vi "X-_Write.vi"(1 "Channel Name":string, 4 "Iteration No":i32, 6 "String to write":string, 7 "Port Name":string, 8 "Value":dbl format="%.2f", 9 "COMMAND":T1, 11 "Address":u8) -> (0 "Good Echo":bool)   [LabVIEW 2010]
uses:
  X-_commands.ctl
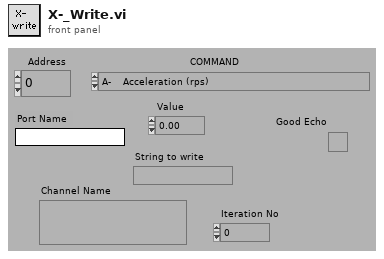
[diagram p1: front panel]
types:
  T1 = typedef "X-_commands.ctl" = enum16{"A-    Acceleration (rps)", "B-    Buffer Status", "C-    Continue", "CG-  Correction Gain", "CR-  Cariage Return", "D-    Distance (pulses)", "DB-  Dead Band (encoder steps)", "DW- Deadband Window (encoder steps)", "E-    Enable Communications", "ER-  Encoder Resolution (steps/rev)", "F-    Disable Communications", "FS-  Encoder Functions Report", "FSA- Incremental/Absolute (0/1)", "FSB- Motor/Encoder Step Mode (0/1)", "FSC- Enable/Disable Position Maint. (1/0)", "FSD- Stop/Continue on Stall (1/0)", "FSE- Activate o/p1 on Stall (1/0)", "FSF- Stop Motion on Trig3 (1/0)", "FSG- Activate o/p2 in Deadband (1/0)", "FSH- Enable Stall Detect (1/0)", "G- Go", "GH- Go Home and Zero (+/-V)", "^H- Delete ", "H- Direction Reverse/CCW/CW (0,1,2)", "IS- Input Status", "K- Kill", "L- Loop (n)", "LD- Limit DISABLE (0-none,1-CW,2-CCW,3-Both)", "LF- Line Feed", "MC- Mode Continuous", "MN- Mode Normal", "MPA- Motor Postion Absolute", "MPI- Motor Position Incremental", "MR- Motor Resolution (Drive Steps/rev)", "N- End of Loop", "O- Output (00,01,10,11)", "OS- Report Homing Setup", "OSA- NO/NC Limits (1/0)", "OSB- Back Up to Home/Edge? (0/1)", "OSC- NO/NC Home Switch (1/0)", "OSD- Enable Encoder Z for Home (0/1)", "OSH- Reference Edge for Home CW/CCW (0/1)", "PR- Report ABSOLUTE Position", "PS- Pause until Continue", "PX- Report Absolute ENCODER Position", "PZ- Zero Absolute Counter", "\"- Quote (17 ASCII +Space)", "Q- Enter/Exit Velocity Profiling (1/0)", "R- Request Indexer Status", "RA- Report Limit Switch Status", "RB- Report Loop, Pause, Shutdown, Trigger Status", "RC- Report Closed Loop Status", "RM- Velocity Streaming Rate Multiplier (000-FFF)", "RV- Report Revision Level", "S- Controlled Stop", "SN- Debounce (1-1000ms)", "SS- Report Software Switch Status", "SSA- Disable RS232 Echo (1/0)", "SSG- Clear/Save Command Buffer on Limit (0/1)", "SSH- Clear/Save Command Buffer on Stop (0/1)", "ST- Shutdown (1/0)", "SV- Servoing Setting (0,1,2,3)", "T- Time Delay (0.01-99999.99)", "TR- Wait for Trigger High/Low/Ignore (1/0/X)", "TS- Report Trigger Status", "U- Pause after Move Until Continue", "V- Velocity (0.01-50.00 revs/sec)", "W1- Report Relative Position <Signed Binary>", "W3- Report Relative Position <Hexadecimal>", "Y- Abort Loop at N", "Z-    Reset to Defaults", "#-    Disable/Set Soft Addresses (0/1-255)"}
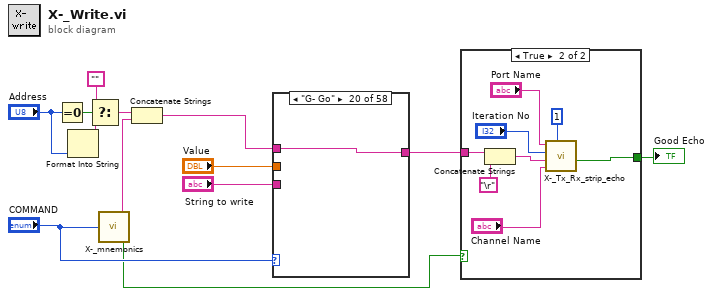
[diagram p0: block diagram]
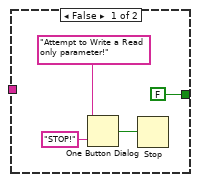
[diagram p2: hidden frame]
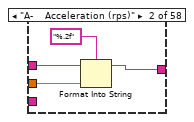
[diagram p4: hidden frame]
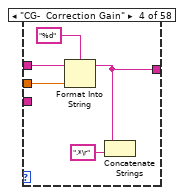
[diagram p6: hidden frame]
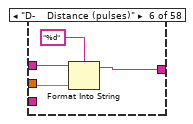
[diagram p8: hidden frame]
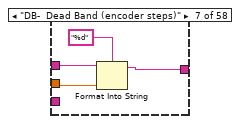
[diagram p9: hidden frame]
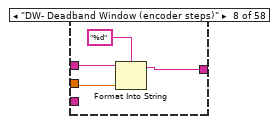
[diagram p10: hidden frame]
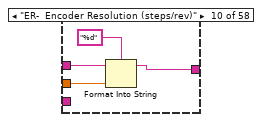
[diagram p12: hidden frame]
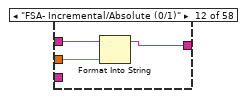
[diagram p14: hidden frame]
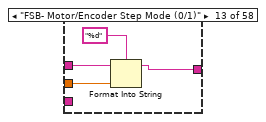
[diagram p15: hidden frame]
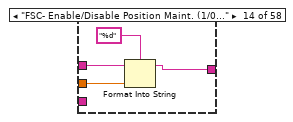
[diagram p16: hidden frame]
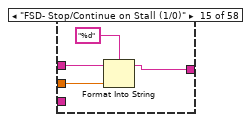
[diagram p17: hidden frame]
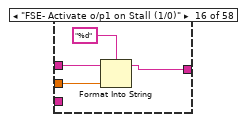
[diagram p18: hidden frame]
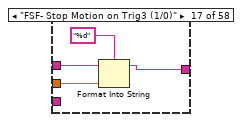
[diagram p19: hidden frame]
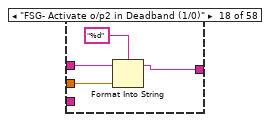
[diagram p20: hidden frame]
diagram:
  n1 = Equal To 0?(x="Address") -> (x = 0?=w8:bool)
  n2 = Format Into String("Address") -> (resulting string=w12:string)  [unwired: 3 in, 1 out]
  n3 = Select(t="", s=w8, f=w12) -> (s? t:f=w13:string)
  n4 = call "X-_mnemonics.vi"("COMMAND"="COMMAND") -> ("Mnemonic"=w3:string, "Writeable"=w2:bool)  [unwired: 1 out]
  n5 = Concatenate Strings(w13, w3) -> (w10:string)
  n6 = case shown="\"G- Go\"" "COMMAND" {
    tunnel: [w14 w15 w19 w22 w25 w28 w32 w36 w38 w41 w43 w44 w48 w52 w56 w60 w64 w68 w72 w75 w77 w79 w82 w84 w85 w88 w90 w91 w92 w93 w94 w96 w99 w101 w105 w110 w114 w118 w122 w124 w125 w128 w132 w136 w138 w142 w146 w150 w154 w158 w162 w166 w169 w171 w177 w179 w180 w183] -> w7
    tunnel: w10 -> [w14 w18 w19 w20 w25 w29 w33 w37 w38 w42 w43 w46 w49 w53 w57 w61 w65 w69 w73 w75 w78 w79 w83 w84 w85 w89 w90 w91 w92 w93 w94 w97 w99 w102 w107 w111 w115 w119 w123 w124 w125 w129 w133 w137 w138 w141 w145 w149 w153 w157 w161 w165 w170 w171 w178 w179 w180 w184]
    tunnel: "Value" -> [_ w17 _ w23 _ w27 w30 w34 _ w40 _ w45 w50 w54 w58 w62 w66 w70 w74 _ w76 _ w81 _ _ w87 _ _ _ _ _ w98 _ w103 w106 w109 w113 w117 w121 _ _ _ w131 w135 _ w140 w144 w148 w152 w156 w160 w164 w168 _ w173 _ _ w182]
    tunnel: "String to write" -> [_ _ _ _ _ _ _ _ _ _ _ _ _ _ _ _ _ _ _ _ _ _ _ _ _ _ _ _ _ _ _ _ _ _ _ _ _ _ _ _ _ w127 _ _ _ _ _ _ _ _ _ _ _ _ _ _ _ _]
    frame Default {
    }
    frame "A-    Acceleration (rps)" {
      n7 = Format Into String(format string="%.2f", initial string=w18, w17) -> (resulting string=w15:string)  [unwired: 1 in, 1 out]
    }
    frame "C-    Continue" {
    }
    frame "CG-  Correction Gain" {
      n8 = Format Into String(format string="%d", initial string=w20, w23) -> (resulting string=w22:string)  [unwired: 1 in, 1 out]
      n9 = Concatenate Strings(w22, ".*\r") -> ()  [unwired: 1 out]
    }
    frame "CR-  Cariage Return" {
    }
    frame "D-    Distance (pulses)" {
      n10 = Format Into String(format string="%d", initial string=w29, w27) -> (resulting string=w28:string)  [unwired: 1 in, 1 out]
    }
    frame "DB-  Dead Band (encoder steps)" {
      n11 = Format Into String(format string="%d", initial string=w33, w30) -> (resulting string=w32:string)  [unwired: 1 in, 1 out]
    }
    frame "DW- Deadband Window (encoder steps)" {
      n12 = Format Into String(format string="%d", initial string=w37, w34) -> (resulting string=w36:string)  [unwired: 1 in, 1 out]
    }
    frame "E-    Enable Communications" {
    }
    frame "ER-  Encoder Resolution (steps/rev)" {
      n13 = Format Into String(format string="%d", initial string=w42, w40) -> (resulting string=w41:string)  [unwired: 1 in, 1 out]
    }
    frame "F-    Disable Communications" {
    }
    frame "FSA- Incremental/Absolute (0/1)" {
      n14 = Format Into String(initial string=w46, w45) -> (resulting string=w44:string)  [unwired: 2 in, 1 out]
    }
    frame "FSB- Motor/Encoder Step Mode (0/1)" {
      n15 = Format Into String(format string="%d", initial string=w49, w50) -> (resulting string=w48:string)  [unwired: 1 in, 1 out]
    }
    frame "FSC- Enable/Disable Position Maint. (1/0)" {
      n16 = Format Into String(format string="%d", initial string=w53, w54) -> (resulting string=w52:string)  [unwired: 1 in, 1 out]
    }
    frame "FSD- Stop/Continue on Stall (1/0)" {
      n17 = Format Into String(format string="%d", initial string=w57, w58) -> (resulting string=w56:string)  [unwired: 1 in, 1 out]
    }
    frame "FSE- Activate o/p1 on Stall (1/0)" {
      n18 = Format Into String(format string="%d", initial string=w61, w62) -> (resulting string=w60:string)  [unwired: 1 in, 1 out]
    }
    frame "FSF- Stop Motion on Trig3 (1/0)" {
      n19 = Format Into String(format string="%d", initial string=w65, w66) -> (resulting string=w64:string)  [unwired: 1 in, 1 out]
    }
    frame "FSG- Activate o/p2 in Deadband (1/0)" {
      n20 = Format Into String(format string="%d", initial string=w69, w70) -> (resulting string=w68:string)  [unwired: 1 in, 1 out]
    }
    frame "FSH- Enable Stall Detect (1/0)" {
      n21 = Format Into String(format string="%d", initial string=w73, w74) -> (resulting string=w72:string)  [unwired: 1 in, 1 out]
    }
    frame "G- Go" {
    }
    frame "GH- Go Home and Zero (+/-V)" {
      n22 = Format Into String(initial string=w78, w76) -> (resulting string=w77:string)  [unwired: 2 in, 1 out]
    }
    frame "^H- Delete " {
    }
    frame "H- Direction Reverse/CCW/CW (0,1,2)" {
      n23 = Pick Line(string ("")=w83, multi-line string="\n-\n+", line index=w81) -> (output string=w82:string)
    }
    frame "K- Kill" {
    }
    frame "L- Loop (n)" {
    }
    frame "LD- Limit DISABLE (0-none,1-CW,2-CCW,3-Both)" {
      n24 = Format Into String(format string="%d", initial string=w89, w87) -> (resulting string=w88:string)  [unwired: 1 in, 1 out]
    }
    frame "LF- Line Feed" {
    }
    frame "MC- Mode Continuous" {
    }
    frame "MN- Mode Normal" {
    }
    frame "MPA- Motor Postion Absolute" {
    }
    frame "MPI- Motor Position Incremental" {
    }
    frame "MR- Motor Resolution (Drive Steps/rev)" {
      n25 = Format Into String(format string="%d", initial string=w97, w98) -> (resulting string=w96:string)  [unwired: 1 in, 1 out]
    }
    frame "N- End of Loop" {
    }
    frame "O- Output (00,01,10,11)" {
      n26 = Format Into String(format string="%2b", initial string=w102, w103) -> (resulting string=w101:string)  [unwired: 1 in, 1 out]
    }
    frame "OSA- NO/NC Limits (1/0)" {
      n27 = Format Into String(format string="%d", initial string=w107, w106) -> (resulting string=w105:string)  [unwired: 1 in, 1 out]
    }
    frame "OSB- Back Up to Home/Edge? (0/1)" {
      n28 = Format Into String(format string="%d", initial string=w111, w109) -> (resulting string=w110:string)  [unwired: 1 in, 1 out]
    }
    frame "OSC- NO/NC Home Switch (1/0)" {
      n29 = Format Into String(format string="%d", initial string=w115, w113) -> (resulting string=w114:string)  [unwired: 1 in, 1 out]
    }
    frame "OSD- Enable Encoder Z for Home (0/1)" {
      n30 = Format Into String(format string="%d", initial string=w119, w117) -> (resulting string=w118:string)  [unwired: 1 in, 1 out]
    }
    frame "OSH- Reference Edge for Home CW/CCW (0/1)" {
      n31 = Format Into String(format string="%d", initial string=w123, w121) -> (resulting string=w122:string)  [unwired: 1 in, 1 out]
    }
    frame "PS- Pause until Continue" {
    }
    frame "PZ- Zero Absolute Counter" {
    }
    frame "\"- Quote (17 ASCII +Space)" {
      n32 = Concatenate Strings(w129, w127, " " ("String to write")) -> (w128:string)
    }
    frame "Q- Enter/Exit Velocity Profiling (1/0)" {
      n33 = Format Into String(format string="%d", initial string=w133, w131) -> (resulting string=w132:string)  [unwired: 1 in, 1 out]
    }
    frame "RM- Velocity Streaming Rate Multiplier (000-FFF)" {
      n34 = Format Into String(format string="%x", initial string=w137, w135) -> (resulting string=w136:string)  [unwired: 1 in, 1 out]
    }
    frame "S- Controlled Stop" {
    }
    frame "SN- Debounce (1-1000ms)" {
      n35 = Format Into String(format string="%d", initial string=w141, w140) -> (resulting string=w142:string)  [unwired: 1 in, 1 out]
    }
    frame "SSA- Disable RS232 Echo (1/0)" {
      n36 = Format Into String(format string="%d", initial string=w145, w144) -> (resulting string=w146:string)  [unwired: 1 in, 1 out]
    }
    frame "SSG- Clear/Save Command Buffer on Limit (0/1)" {
      n37 = Format Into String(format string="%d", initial string=w149, w148) -> (resulting string=w150:string)  [unwired: 1 in, 1 out]
    }
    frame "SSH- Clear/Save Command Buffer on Stop (0/1)" {
      n38 = Format Into String(format string="%d", initial string=w153, w152) -> (resulting string=w154:string)  [unwired: 1 in, 1 out]
    }
    frame "ST- Shutdown (1/0)" {
      n39 = Format Into String(format string="%d", initial string=w157, w156) -> (resulting string=w158:string)  [unwired: 1 in, 1 out]
    }
    frame "SV- Servoing Setting (0,1,2,3)" {
      n40 = Format Into String(format string="%d", initial string=w161, w160) -> (resulting string=w162:string)  [unwired: 1 in, 1 out]
    }
    frame "T- Time Delay (0.01-99999.99)" {
      n41 = Format Into String(format string="%.2f", initial string=w165, w164) -> (resulting string=w166:string)  [unwired: 1 in, 1 out]
    }
    frame "TR- Wait for Trigger High/Low/Ignore (1/0/X)" {
      n42 = Pick Line(string ("")=w170, multi-line string="0\n1\nX", line index=w168) -> (output string=w169:string)
    }
    frame "U- Pause after Move Until Continue" {
    }
    frame "V- Velocity (0.01-50.00 revs/sec)" {
      w174 = 0.0  # Min
      w175 = 50.0  # Max
      n43 = In Range and Coerce(upper limit=w175, x=w173, lower limit=w174) -> (coerced(x)=w172:dbl)  [unwired: 1 out]
      n44 = Format Into String(format string="%.2f", initial string=w178, w172) -> (resulting string=w177:string)  [unwired: 1 in, 1 out]
    }
    frame "Y- Abort Loop at N" {
    }
    frame "Z-    Reset to Defaults" {
    }
    frame "#-    Disable/Set Soft Addresses (0/1-255)" {
      n45 = Format Into String(format string="%d", initial string=w184, w182) -> (resulting string=w183:string)  [unwired: 1 in, 1 out]
    }
  }
  n46 = case shown="True" w2 {
    tunnel: w7 -> [_ w196]
    tunnel: [FALSE ("Good Echo") w191] -> w1
    frame False {
      n47 = One Button Dialog(message="Attempt to Write a Read only parameter!", button name ("OK")="STOP!") -> (true=w186:bool)
      n48 = Stop(stop? (T)=w186) -> ()
    }
    frame True {
      n49 = Concatenate Strings(w196, "\r") -> (w195:string)
      n50 = call "X-_Tx_Rx_strip_echo.vi"("Terminate Count"=1, "Channel Name"="Channel Name", "Write String"=w195, "Iteration No"="Iteration No", "Port Name"="Port Name") -> ("Good Echo"=w191:bool)  [unwired: 3 out]
    }
  }
  "Good Echo" <- w1
